vi "temp_avi.vi"() -> ()   [LabVIEW 2018]
doc: "This example performs writes and reads on a serial port, as directed by the user. You can press the Write and Read buttons, and change the Read Count, while the example is running.\n\nThe parameters set for the serial port must match the parameters of the connected instrument or device. In this example, the Read Count parameter specifies the number of bytes that the serial port reads. If there were more bytes at the port than the specified number, those bytes would not be read. If there were less bytes at the port than the specified number, you would receive a timeout error.\n\nThis example expands upon the flow control options for XON and XOFF, allowing the user to choose those control characters. Also, the user can enable or disable a termination character. Some devices require a termination character in order to identify the end of command strings. Some devices send a termination character to signify the end of data to be read. This example shows how you can end the Read operation once a termination character is detected in the buffer and/or append a termination character at the end of the Write data."
uses:
  <vilib>/Instr/_visa.llb/VISA Configure Serial Port (Instr).vi
panel:
  out "최대온도":dbl
  out "웨이브폼 차트":dbl(graph)
  in  "Frames Per Second":u32=10
  in  "AVI Path":path=path "E:/temp/b.avi"
  in  "stop 4":bool
  in  "stop 3":bool
  in  "폭":dbl=10.0
  in  "중심":dbl=35.0
  out "Temperature":dbl[][](graph)
  in  "Stop":bool
  in  "VISA resource name":refnum<visa-resource-name>="COM6"
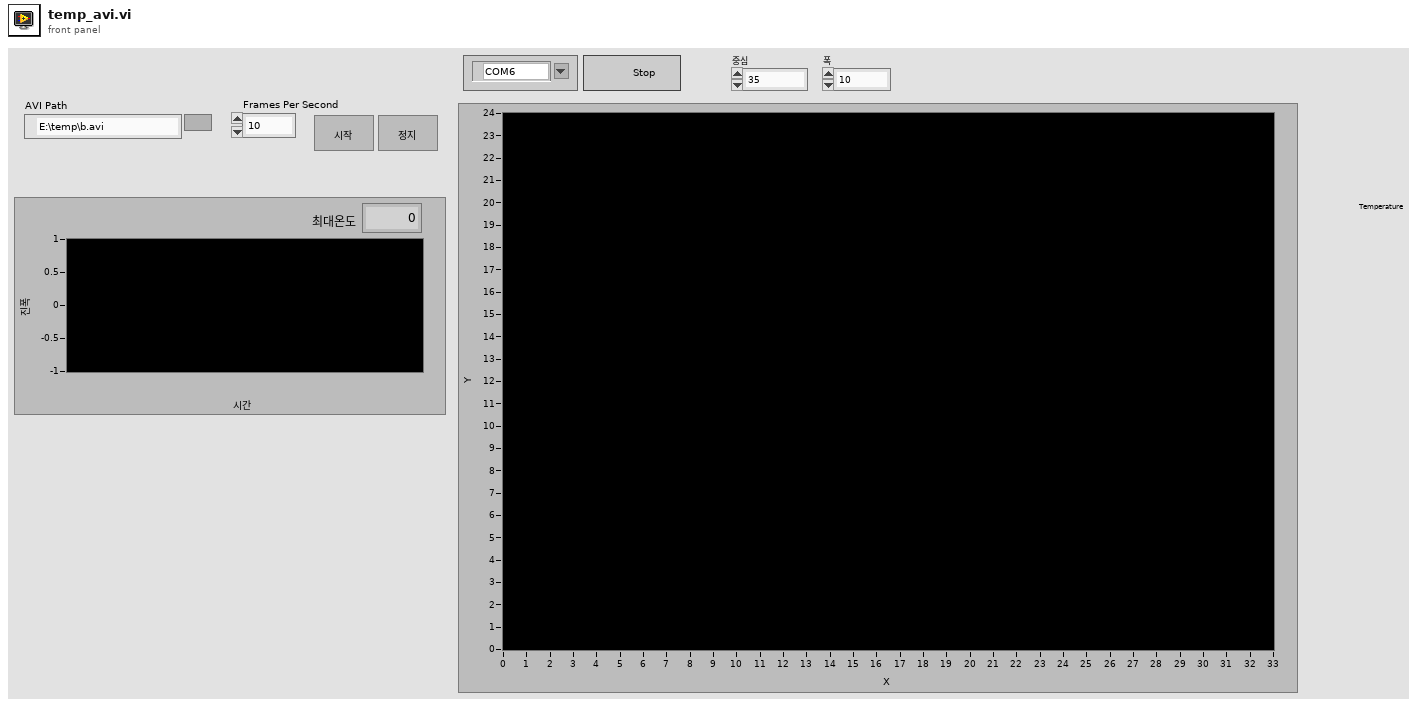
[diagram p1: front panel]
types:
  T1 = typedef "Image Type" = u32
  T2 = typedef "IMAQ Image.ctl" = refnum<image>
  T3 = typedef "IMAQ AVI2 Refnum.ctl" = refnum<k20>
  T4 = typedef "imagedata.ctl" = cluster{"image type":i32, "image depth":i32, "image":u8[], "mask":u8[], "colors":u32[], "Rectangle":cluster{"left":i16, "top":i16, "right":i16, "bottom":i16}}
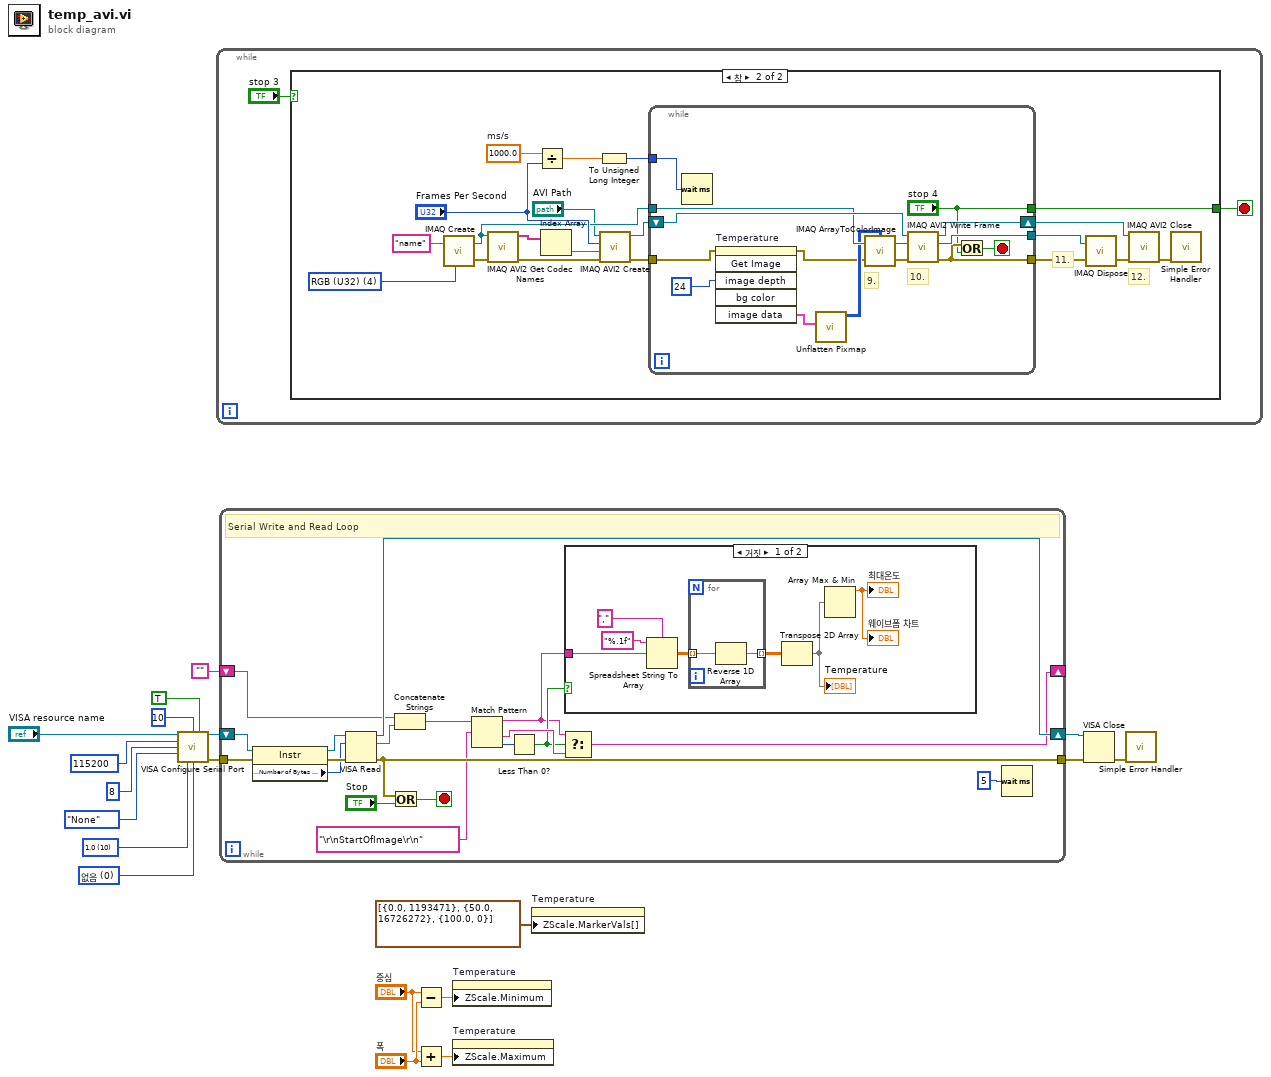
[diagram p0: block diagram]
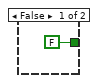
[diagram p2: hidden frame]
diagram:
  w6 = u16 0 items=["없음", "XON/XOFF", "RTS/CTS", "XON/XOFF & RTS/CTS", "DTR/DSR", "XON/XOFF & DTR/DSR"] ("flow control (0:none)")
  w7 = u16 10 items=["1.0"=10, "1.5"=15, "2.0"=20] ("stop bits (10: 1 bit)")
  n1 = call-poly "VISA Configure Serial Port"("VISA resource name"="VISA resource name", "termination char\n(0xA = '\\n' = LF)"=u8 10 ("Termination Character"), "Enable Termination\nChar (T)"=TRUE ("End Read on Termination Character?"), "baud rate (9600)"=u32 115200, "data bits (8)"=u16 8, "parity (0:none)"=enum16{"None", "Odd", "Even", "Mark", "Space"}."None", "stop bits (10: 1 bit)"=w7, "flow control (0:none)"=w6) -> ("VISA resource name out"=w13:refnum<visa-resource-name>, "error out"=w12:errorcluster)  [unwired: 2 in, 4 out]
  n2 = while {
    stop <- w20 stop-if-true
    n3 = case shown="참" "stop 3" {
      tunnel: [FALSE ("stop") w23] -> w20
      frame False {
      }
      frame True {
        w26 = 1000.0  # ms/s
        w24 = T1 4 items=["Grayscale (U8)", "Grayscale (I16)", "Grayscale (SGL)", "Complex (CSG)", "RGB (U32)", "HSL (U32)", "RGB (U64)", "Grayscale (U16)"] ("Image Type")
        # "12."
        # "11."
        n4 = call "IMAQ Create"("Image Name"="name", "Image Type"=w24) -> ("New Image"=w36:T2, "error out"=w35:errorcluster)  [unwired: 3 in]
        n5 = call "IMAQ AVI2 Get Codec Names"("error in (no error)"=w35, "Image"=w36) -> ("error out"=w34:errorcluster, "Codec Names"=w38:string[])  [unwired: 8 in]
        n6 = Divide(x=w26, y="Frames Per Second") -> (x/y=w41:dbl)
        n7 = Index Array(array=w38) -> (element=w39:string)  [unwired: 1 in]
        n8 = To Unsigned Long Integer(number=w41) -> (unsigned 32bit integer=w42:u32)
        n9 = call "IMAQ AVI2 Create"("error in (no error)"=w34, "Codec"=w39, "Frames Per Second"="Frames Per Second", "AVI Path"="AVI Path") -> ("error out"=w37:errorcluster, "AVI Refnum"=w33:T3)  [unwired: 6 in]
        n10 = while {
          tunnel: w36 -> [w51]
          tunnel: w37 -> [w45]
          tunnel: [w55] -> w27
          tunnel: [w52] -> w28
          shift-right: [w56] -> w29
          shift-left: w33 -> [w57]
          tunnel: w42 -> [w54]
          tunnel: ["stop 4"] -> w23
          stop <- w53 stop-if-true
          # "10."
          # "9."
          n11 = Wait (ms)(milliseconds to wait=w54) -> ()  [unwired: 1 out]
          n12 = invoke on="Temperature" class="IntGraph (엄격한)" method="Get Image"(error in=w45, "image depth"=24 ("Image Depth")) -> (error out=w44:errorcluster, "image data"=w46:T4)  [unwired: 4 in, 4 out]
          n13 = call <vilib>:"Unflatten Pixmap.vi"("image data"=w46) -> ("24-bit pixmap"=w48:u32[][])  [unwired: 4 in, 6 out]
          n14 = call "IMAQ ArrayToColorImage"("Image Pixels (U32)"=w48, "Image"=w51, "error in (no error)"=w44) -> ("Image Out"=w50:T2, "error out"=w49:errorcluster)  [unwired: 2 in]
          n15 = call "IMAQ AVI2 Write Frame"("error in (no error)"=w49, "Image"=w50, "AVI Refnum"=w57) -> ("error out"=w52:errorcluster, "Image Out (duplicate)"=w55:T2, "AVI Refnum (duplicate)"=w56:T3)  [unwired: 6 in]
          n16 = Or(x=w52, y="stop 4") -> (x .or. y?=w53:bool)
        }
        n17 = call "IMAQ Dispose"("Image"=w27, "error in (no error)"=w28) -> ("error out"=w30:errorcluster)  [unwired: 4 in]
        n18 = call "IMAQ AVI2 Close"("error in (no error)"=w30, "AVI Refnum"=w29) -> ("error out"=w31:errorcluster)  [unwired: 9 in]
        n19 = call <vilib>:"Simple Error Handler.vi"("error in (no error)"=w31) -> ()  [unwired: 4 in, 5 out]
      }
    }
  }
  n20 = while {
    shift-right: [w71] -> w15
    shift-left: w13 -> [w73]
    tunnel: w12 -> [w69]
    tunnel: [w65] -> w16
    shift-right: [w58] -> _
    shift-left: "" -> [w67]
    stop <- w75 stop-if-true
    # "Serial Write and Read Loop"
    n21 = property class="Instr"(reference=w73, error in=w69) -> (reference out=w72:refnum<visa-resource-name>, error out=w70:errorcluster, "Serial Settings:Number of Bytes at Serial Port"=w68:u32)
    n22 = VISA Read(VISA resource name=w72, byte count=w68, error in (no error)=w70) -> (VISA resource name out=w71:refnum<visa-resource-name>, read buffer=w66:string, error out=w65:errorcluster)  [unwired: 1 out]
    n23 = Or(x=w65, y="Stop") -> (x .or. y?=w75:bool)
    n24 = Concatenate Strings(w67, w66) -> (w63:string)
    n25 = Match Pattern(string=w63, regular expression="\r\nStartOfImage\r\n") -> (before substring=w59:string, after substring=w61:string, offset past match=w62:i32)  [unwired: 1 in, 1 out]
    n26 = Less Than 0?(x=w62) -> (x < 0?=w60:bool)
    n27 = Select(t=w59, s=w60, f=w61) -> (s? t:f=w58:string)
    n28 = case shown="거짓" w60 {
      tunnel: w59 -> [w82 _]
      frame False {
        n29 = Spreadsheet String To Array(delimiter (Tab)=",", format string="%.1f", spreadsheet string=w82) -> (array=w80:dbl[][])  [unwired: 1 in]
        n30 = for {
          tunnel: w80 -> [w85] mode=indexing
          tunnel: [w84] -> w79 mode=indexing
          n31 = Reverse 1D Array(array=w85) -> (reversed array=w84:dbl[])
        }
        n32 = Transpose 2D Array(2D array=w79) -> (transposed array=w77:dbl[][])
        "Temperature" <- w77
        n33 = Array Max & Min(array=w77) -> (max value=→"최대온도" →"웨이브폼 차트":dbl)  [unwired: 3 out]
      }
      frame True {
      }
    }
    n34 = Wait (ms)(milliseconds to wait=u32 5) -> ()  [unwired: 1 out]
  }
  n35 = Subtract(x="중심", y="폭") -> (x-y=w5:dbl)
  n36 = Add(x="중심", y="폭") -> (x+y=w1:dbl)
  n37 = property on="Temperature" class="IntGraph (엄격한)"("ZScale.Minimum"=w5) -> ()  [unwired: 2 in, 2 out]
  n38 = property on="Temperature" class="IntGraph (엄격한)"("ZScale.Maximum"=w1) -> ()  [unwired: 2 in, 2 out]
  n39 = property on="Temperature" class="IntGraph (엄격한)"("ZScale.MarkerVals[]"=cluster{dbl, u32}[] [{0.0, 1193471}, {50.0, 16726272}, {100.0, 0}] ("Z 스케일.마커 값[]")) -> ()  [unwired: 2 in, 2 out]
  n40 = VISA Close(VISA resource name=w15, error in (no error)=w16) -> (error out=w17:errorcluster)
  n41 = call <vilib>:"Simple Error Handler.vi"("error in (no error)"=w17) -> ()  [unwired: 1 in, 8 out]
